vi "Data Storage.vi"(9 "Time Out In ms":i32=-1, 10 "Data In":u16[](array[numeric]), 11 "Circular Buffer 1D U16 DVR Queue in":refnum<class "Circular Buffer 1D U16 DVR Queue.lvclass">) -> (1 "Time Out":bool, 3 "Circular Buffer 1D U16 DVR Queue out":refnum<class "Circular Buffer 1D U16 DVR Queue.lvclass">)   [LabVIEW 2024, in "Circular Buffer 1D U16 DVR Queue.lvclass"]
uses:
  Circular Buffer 1D U16 DVR Queue.lvclass
  Circular Buffer 1D U16 DVR Queue.lvclass/Circular Buffer 1D U16 DVR Queue.ctl
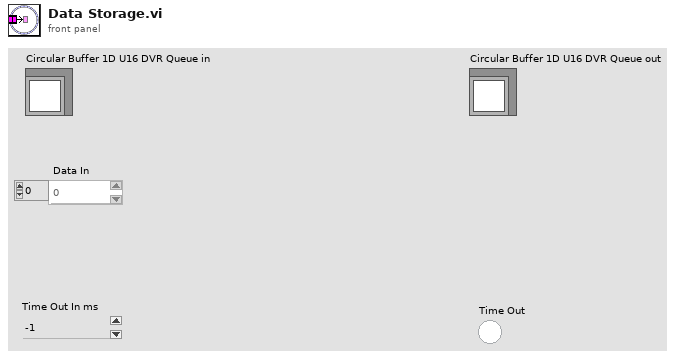
[diagram p1: front panel]
types:
  T1 = typedef "1D U16 DVR Queue.ctl" = refnum<queue>
  T2 = typedef "1D U16 DVR.ctl" = refnum<data-value>
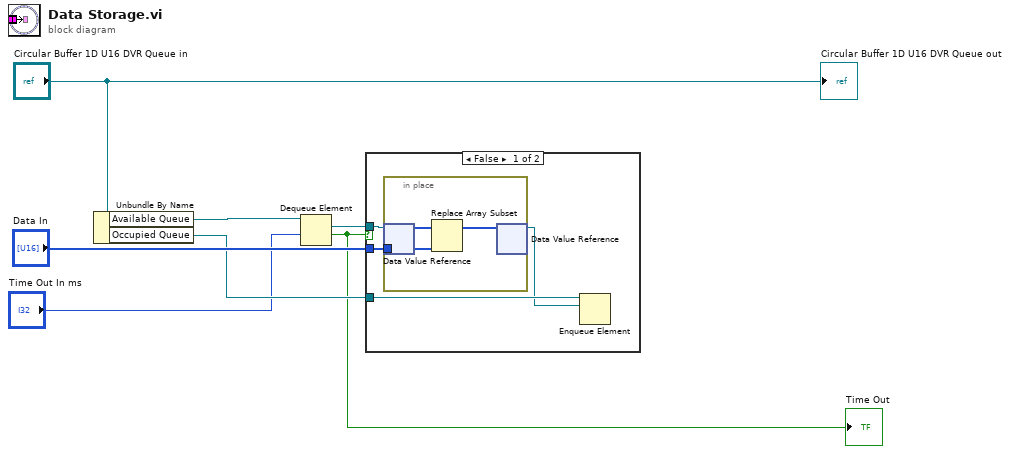
[diagram p0: block diagram]
diagram:
  n1 = Unbundle By Name("Circular Buffer 1D U16 DVR Queue in") -> ("Available Queue"=w4:T1, "Occupied Queue"=w5:T1)
  n2 = Dequeue Element(queue=w4, timeout in ms (-1)="Time Out In ms") -> (element=w2:T2, timed out?=w1:bool)  [unwired: 1 in, 2 out]
  "Time Out" <- w1
  n3 = case shown="False" w1 {
    tunnel: "Data In" -> [w11 _]
    tunnel: w2 -> [w10 _]
    tunnel: w5 -> [w9 _]
    frame False {
      n4 = in-place {
        in-place-border: w11 -> [w12]
        n5 = in-place-dvr #1(w10) -> (w14:u16[])  [unwired: 1 out]
        n6 = Replace Array Subset(array=w14, new element=w12) -> (w13:u16[])  [unwired: 1 in]
        n7 = in-place-dvr #1(w13) -> (w8:T2)  [unwired: 1 out]
      }
      n8 = Enqueue Element(queue=w9, element=w8) -> ()  [unwired: 2 in, 3 out]
    }
    frame True {
    }
  }
  "Circular Buffer 1D U16 DVR Queue out" <- "Circular Buffer 1D U16 DVR Queue in"
